vi "Send D0.vi"(8 "error in (no error)":errorcluster, 11 "H3611i Actor in":refnum<class "H3611i Actor.lvclass">) -> (0 "error out":errorcluster, 2 "Range":string, 3 "H3611i Actor out":refnum<class "H3611i Actor.lvclass">)   [LabVIEW 2018, in "H3611i.lvlib" / "H3611i Actor.lvclass"]
uses:
  H3611i Actor.lvclass
  C:/Users/dev/Documents/CODE/LabVIEW/microwaveverify/trunk/MWWL Verification/Sensor Actor/Sensor/Sensor.lvclass
  H3611i Actor.lvclass/H3611i Actor.ctl
  Sensor Actor/Sensor/Sensor.lvclass
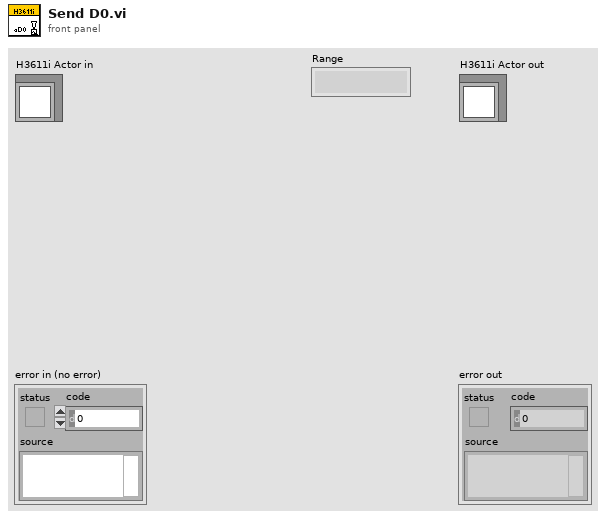
[diagram p1: front panel]
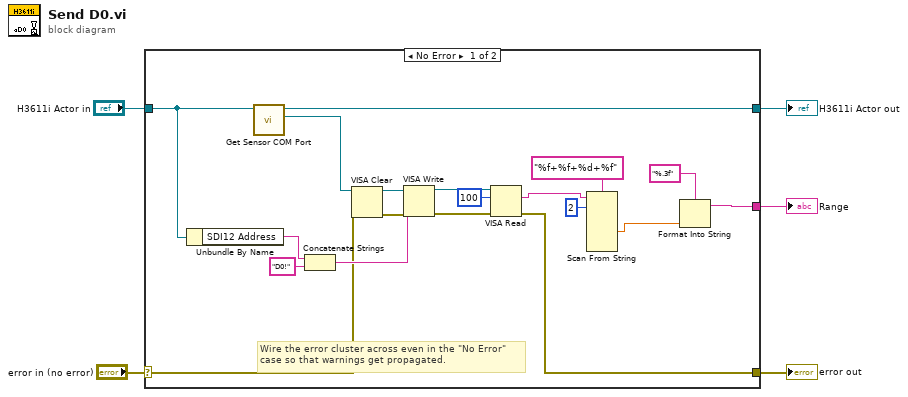
[diagram p0: block diagram]
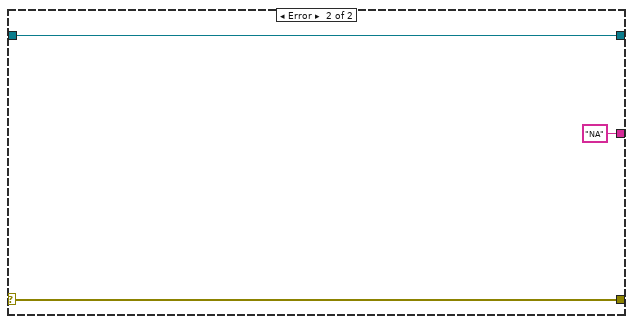
[diagram p2: hidden frame]
diagram:
  n1 = case shown="No Error" "error in (no error)" {
    selector: "error in (no error)" -> [w15 w27]
    tunnel: [w19 w27] -> w4
    tunnel: [w12 w26] -> w2
    tunnel: "H3611i Actor in" -> [w24 w26]
    tunnel: [w7 "NA"] -> w1
    frame No Error {
      # "Wire the error cluster across even in the \"No Error\"\ncase so that warnings get propagated."
      n2 = Unbundle By Name(w24) -> ("SDI12 Address"=w23:string)
      n3 = call "Get Sensor COM Port.vi"("Sensor in"=w24) -> ("COM Port"=w16:refnum<visa-resource-name>, "Sensor out"=w12:refnum<class "H3611i Actor.lvclass">)  [unwired: 8 in, 1 out]
      n4 = Concatenate Strings(w23, "D0!" ("string")) -> (w21:string)
      n5 = VISA Clear(VISA resource name=w16, error in (no error)=w15) -> (VISA resource name out=w13:refnum<visa-resource-name>, error out=w14:errorcluster)
      n6 = VISA Write(VISA resource name=w13, write buffer=w21, error in (no error)=w14) -> (VISA resource name out=w18:refnum<visa-resource-name>, error out=w20:errorcluster)  [unwired: 1 out]
      n7 = VISA Read(VISA resource name=w18, byte count=u32 100, error in (no error)=w20) -> (read buffer=w9:string, error out=w19:errorcluster)  [unwired: 2 out]
      n8 = Scan From String(format string="%f+%f+%d+%f", input string=w9, initial scan location=u32 2) -> (output 2=w6:dbl)  [unwired: 8 in, 3 out]
      n9 = Format Into String(format string="%.3f", w6) -> (resulting string=w7:string)  [unwired: 2 in, 1 out]
    }
    frame Error {
    }
  }
  "error out" <- w4
  "H3611i Actor out" <- w2
  "Range" <- w1
